vi "ConnToMasterErr.vi"(11 "String":string) -> (3 "Abort?":bool)   [LabVIEW 2012]
uses:
  <vilib>/Platform/browser.llb/Open URL in Default Browser (string).vi
panel:
  in  "OK Button":bool
  in  "Website":bool
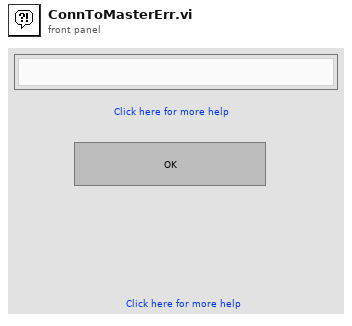
[diagram p1: front panel]
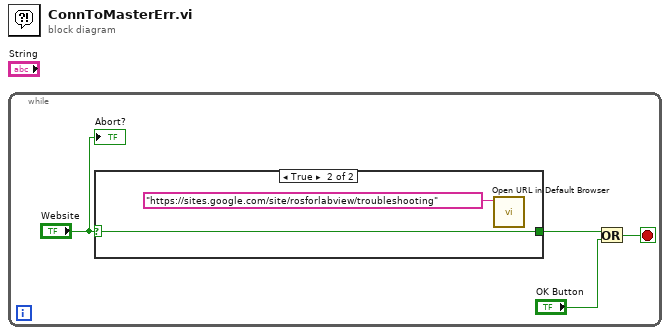
[diagram p0: block diagram]
diagram:
  n1 = while {
    stop <- w1 stop-if-true
    n2 = case shown="True" "Website" {
      selector: "Website" -> [_ w6]
      tunnel: [_ w6] -> w2
      frame False {
      }
      frame True {
        n3 = call-poly <vilib>:"Open URL in Default Browser.vi"("URL"="https://sites.google.com/site/rosforlabview/troubleshooting") -> ()  [unwired: 5 in, 2 out]
      }
    }
    n4 = Or(x=w2, y="OK Button") -> (x .or. y?=w1:bool)
    "Abort?" <- "Website"
  }
